vi "棋盘初始化.vi"() -> (0 "游戏":T1)   [LabVIEW 2017]
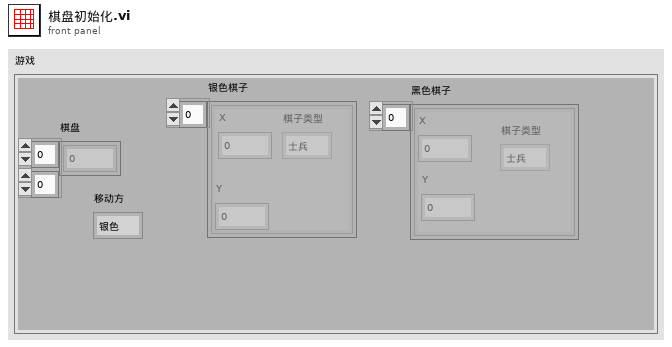
[diagram p1: front panel]
types:
  T1 = cluster{"棋盘":u16[][], "银色棋子":cluster{"棋子类型":enum16{"士兵", "骑士", "主教", "战车", "皇后", "国王", "空"}, "X":u8, "Y":u8}[], "黑色棋子":cluster{"棋子类型":enum16{"士兵", "骑士", "主教", "战车", "皇后", "国王", "空"}, "X":u8, "Y":u8}[], "移动方":enum16{"银色", "黑色"}}
  T2 = cluster{"棋子类型":enum16{"士兵", "骑士", "主教", "战车", "皇后", "国王", "空"}, u8, u8}[]
  T3 = cluster{"棋子类型":enum16{"士兵", "骑士", "主教", "战车", "皇后", "国王", "空"}, u8, u8}
  T4 = cluster{u16[][], cluster{"棋子类型":enum16{"士兵", "骑士", "主教", "战车", "皇后", "国王", "空"}, u8, u8}[], cluster{"棋子类型":enum16{"士兵", "骑士", "主教", "战车", "皇后", "国王", "空"}, u8, u8}[], enum16{"银色", "黑色"}}
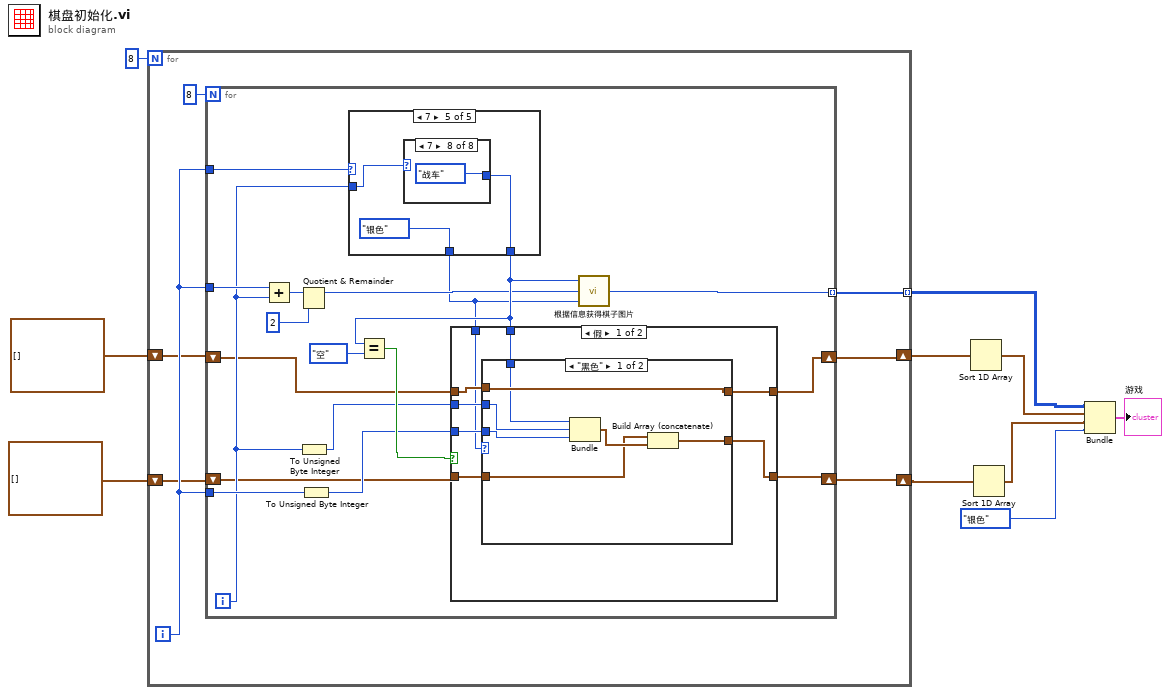
[diagram p0: block diagram]
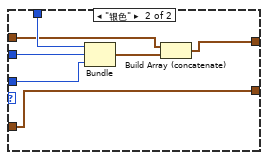
[diagram p2: hidden frame]
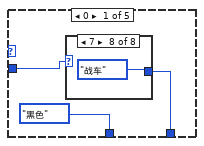
[diagram p4: hidden frame]
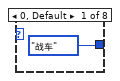
[diagram p5: hidden frame]
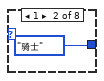
[diagram p6: hidden frame]
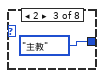
[diagram p7: hidden frame]
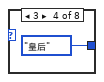
[diagram p8: hidden frame]
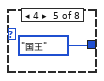
[diagram p9: hidden frame]
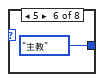
[diagram p10: hidden frame]
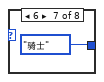
[diagram p11: hidden frame]
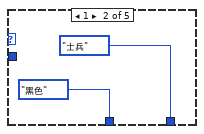
[diagram p12: hidden frame]
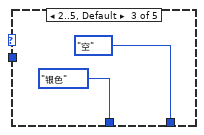
[diagram p13: hidden frame]
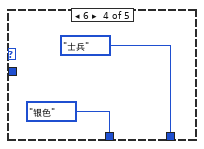
[diagram p14: hidden frame]
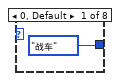
[diagram p15: hidden frame]
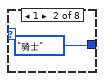
[diagram p16: hidden frame]
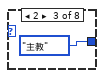
[diagram p17: hidden frame]
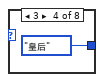
[diagram p18: hidden frame]
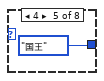
[diagram p19: hidden frame]
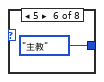
[diagram p20: hidden frame]
diagram:
  n1 = for {
    N: 8 -> [_]
    shift-right: [w14] -> w9
    shift-left: T2 [] -> [w15]
    tunnel: [w13] -> w8 mode=indexing
    shift-right: [w11] -> w4
    shift-left: T2 [] -> [w12]
    i -> [w16]
    n2 = for {
      N: 8 -> [_]
      tunnel: w16 -> [w35]
      tunnel: w16 -> [w34]
      tunnel: w16 -> [w30]
      shift-right: [w27] -> w14
      shift-left: w15 -> [w28]
      tunnel: [w21] -> w13 mode=indexing
      shift-right: [w18] -> w11
      shift-left: w12 -> [w19]
      i -> [w29]
      n3 = Add(x=w34, y=w29) -> (x+y=w33:i32)
      n4 = Quotient & Remainder(x=w33, y=2) -> (x-y*floor(x/y)=w23:i32)  [unwired: 1 out]
      n5 = To Unsigned Byte Integer(number=w29) -> (unsigned 8bit integer=w26:u8)
      n6 = To Unsigned Byte Integer(number=w30) -> (unsigned 8bit integer=w25:u8)
      n7 = case shown="7" w35 {
        tunnel: w29 -> [w62 _ _ _ w78]
        tunnel: [w61 enum16{"士兵", "骑士", "主教", "战车", "皇后", "国王", "空"}."士兵" ("棋子类型") enum16{"士兵", "骑士", "主教", "战车", "皇后", "国王", "空"}."空" ("棋子类型") enum16{"士兵", "骑士", "主教", "战车", "皇后", "国王", "空"}."士兵" ("棋子类型") w77] -> w24
        tunnel: [enum16{"银色", "黑色"}."黑色" enum16{"银色", "黑色"}."黑色" enum16{"银色", "黑色"}."银色" enum16{"银色", "黑色"}."银色" enum16{"银色", "黑色"}."银色"] -> w22
        frame 0 {
          n8 = case shown="7" w62 {
            tunnel: [enum16{"士兵", "骑士", "主教", "战车", "皇后", "国王", "空"}."战车" ("棋子类型") enum16{"士兵", "骑士", "主教", "战车", "皇后", "国王", "空"}."骑士" ("棋子类型") enum16{"士兵", "骑士", "主教", "战车", "皇后", "国王", "空"}."主教" ("棋子类型") enum16{"士兵", "骑士", "主教", "战车", "皇后", "国王", "空"}."皇后" ("棋子类型") enum16{"士兵", "骑士", "主教", "战车", "皇后", "国王", "空"}."国王" ("棋子类型") enum16{"士兵", "骑士", "主教", "战车", "皇后", "国王", "空"}."主教" ("棋子类型") enum16{"士兵", "骑士", "主教", "战车", "皇后", "国王", "空"}."骑士" ("棋子类型") enum16{"士兵", "骑士", "主教", "战车", "皇后", "国王", "空"}."战车" ("棋子类型")] -> w61
            frame 0, Default {
            }
            frame 1 {
            }
            frame 2 {
            }
            frame 3 {
            }
            frame 4 {
            }
            frame 5 {
            }
            frame 6 {
            }
            frame 7 {
            }
          }
        }
        frame 1 {
        }
        frame 2..5, Default {
        }
        frame 6 {
        }
        frame 7 {
          n9 = case shown="7" w78 {
            tunnel: [enum16{"士兵", "骑士", "主教", "战车", "皇后", "国王", "空"}."战车" ("棋子类型") enum16{"士兵", "骑士", "主教", "战车", "皇后", "国王", "空"}."骑士" ("棋子类型") enum16{"士兵", "骑士", "主教", "战车", "皇后", "国王", "空"}."主教" ("棋子类型") enum16{"士兵", "骑士", "主教", "战车", "皇后", "国王", "空"}."皇后" ("棋子类型") enum16{"士兵", "骑士", "主教", "战车", "皇后", "国王", "空"}."国王" ("棋子类型") enum16{"士兵", "骑士", "主教", "战车", "皇后", "国王", "空"}."主教" ("棋子类型") enum16{"士兵", "骑士", "主教", "战车", "皇后", "国王", "空"}."骑士" ("棋子类型") enum16{"士兵", "骑士", "主教", "战车", "皇后", "国王", "空"}."战车" ("棋子类型")] -> w77
            frame 0, Default {
            }
            frame 1 {
            }
            frame 2 {
            }
            frame 3 {
            }
            frame 4 {
            }
            frame 5 {
            }
            frame 6 {
            }
            frame 7 {
            }
          }
        }
      }
      n10 = Equal?(x=w24, y=enum16{"士兵", "骑士", "主教", "战车", "皇后", "国王", "空"}."空") -> (x = y?=w31:bool)
      n11 = case shown="假" w31 {
        tunnel: [w39 w59] -> w27
        tunnel: w28 -> [w40 w59]
        tunnel: w19 -> [w36 w58]
        tunnel: [w37 w58] -> w18
        tunnel: w26 -> [w42 _]
        tunnel: w25 -> [w41 _]
        tunnel: w24 -> [w43 _]
        tunnel: w22 -> [w38 _]
        frame False {
          n12 = case shown="\"黑色\"" w38 {
            tunnel: w43 -> [w49 w57]
            tunnel: w42 -> [w48 w56]
            tunnel: w41 -> [w47 w55]
            tunnel: w40 -> [w50 w54]
            tunnel: [w50 w52] -> w39
            tunnel: w36 -> [w44 w51]
            tunnel: [w45 w51] -> w37
            frame "黑色" {
              n13 = Bundle("棋子类型"=w49, w48, w47) -> (w46:T3)  [unwired: 1 in]
              n14 = Build Array (concatenate)(w44, w46) -> (w45:T2)
            }
            frame "银色" {
              n15 = Bundle("棋子类型"=w57, w56, w55) -> (w53:T3)  [unwired: 1 in]
              n16 = Build Array (concatenate)(w54, w53) -> (w52:T2)
            }
          }
        }
        frame True {
        }
      }
      n17 = call "根据信息获得棋子图片.vi"("棋子颜色"=w22, "背景颜色"=w23, "棋子类型"=w24) -> ("棋子"=w21:u16)
    }
  }
  n18 = Sort 1D Array(array=w9) -> (sorted array=w5:T2)
  n19 = Sort 1D Array(array=w4) -> (sorted array=w7:T2)
  n20 = Bundle(w8, w5, w7, enum16{"银色", "黑色"}."银色") -> (→"游戏":T4)  [unwired: 1 in]
